vi "Remove Clients.vi"(8 "error in (no error)":errorcluster, 10 "Client":string, 11 "Server Client in":refnum<class "Server Client.lvclass">) -> (0 "error out":errorcluster, 3 "Server Client out":refnum<class "Server Client.lvclass">)   [LabVIEW 2020, in "Server Client.lvclass"]
uses:
  Server Client.lvclass
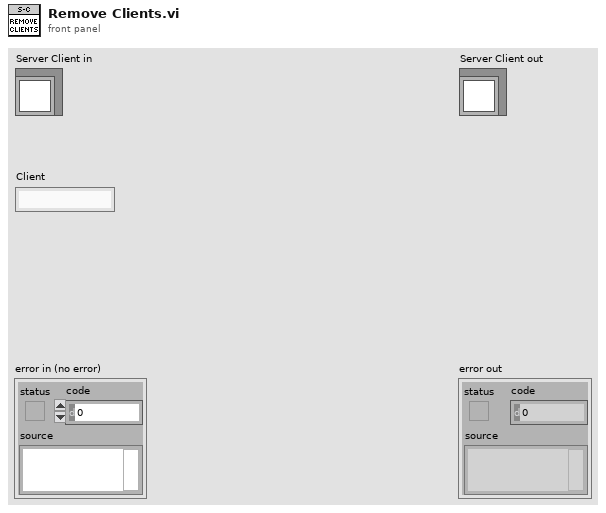
[diagram p1: front panel]
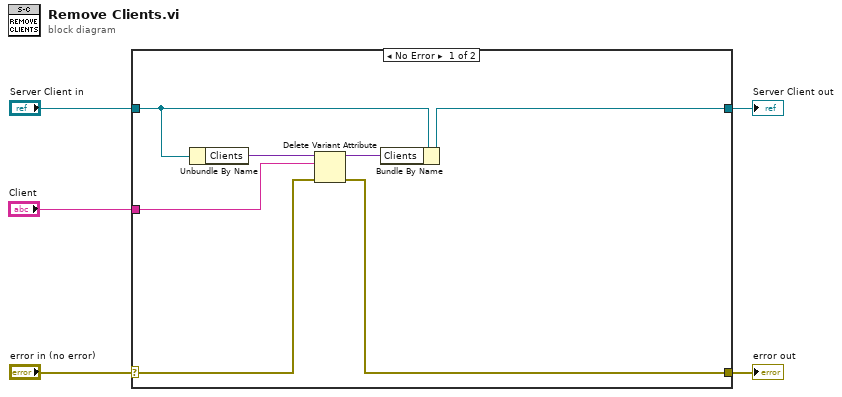
[diagram p0: block diagram]
diagram:
  n1 = case shown="No Error" "error in (no error)" {
    selector: "error in (no error)" -> [w9 w14]
    tunnel: [w6 w14] -> w4
    tunnel: [w8 w13] -> w2
    tunnel: "Server Client in" -> [w12 w13]
    tunnel: "Client" -> [w10 _]
    frame No Error {
      n2 = Unbundle By Name(w12) -> ("Clients"=w11:variant)
      n3 = Delete Variant Attribute(4:w9, 6:w10, 7:w11) -> (0:w6:errorcluster, 3:w7:variant)  [unwired: 1 out]
      n4 = Bundle By Name(cluster=w12, "Clients"=w7) -> (w8:refnum<class "Server Client.lvclass">)
    }
    frame Error {
    }
  }
  "error out" <- w4
  "Server Client out" <- w2
